vi "SPCSplitIntensityFrames.vi"(6 "New Image Size\nwhen != 0":T1={"X Size"=0, "Y Size"=0, "adc_res"=4096, "NoOfRoutingChannel"=1}, 8 "Error In":errorcluster, 9 "SPC/QC":bool=TRUE, 10 "EventData":u16[](array[numeric]) format="%04x", 11 "ROIShifts":cluster{dbl, dbl}[](array[cluster])) -> (0 "Error Out":errorcluster, 1 "IntensityFrames":cluster{u32[][]}[](array[cluster]), 2 "AbsoluteIntensity":u32[](array[numeric]), 3 "DecayMatrix":u16[][][][](array[numeric]), 4 "FrameEvents":i32[](array[numeric]), 5 "IntensityGraph":u32[][](graph), 7 "MaxIntensity":u32)   [LabVIEW 2019]
doc: "This VI goes through an EventData-Array received from 'SPC_read_fifo.vi' and interprets the events as markers or photons and populates a DecayMatrix for a single frame.\nThe 4 dimensions of DecayMatrix are the decay curves according to the microTime values of photons, in their image X- and Y-axis position and routing channel.\nNote the two possible ways of creating an IntensityGraph: With every photon event the intensity could increase per X-Y-coordinate, or the really counted photon number during a pixel event is used (usually higher).\nA functional global variable concept is used to initialize the control cluster and output arrays.\nThis VI accumulates only events for one frame.\nA similar VI used at the executable example 'ImagingEventStream-FifoImage.exe' that also collects multiple frames with improved memory management is available at B&H.\n\ninfo@becker-hickl.com"
uses:
  SPC_Controls/Fifo_CounterCluster.ctl
panel:
  out "BufferedImageSize":T1={"X Size"=0, "Y Size"=0, "adc_res"=0, "NoOfRoutingChannel"=1}
  out "CounterCluster":T2={"Pixel No"=0, "Frame No"=-1, "LastPixelTime"=0, "Line No"=-1, "StopFrame"=FALSE, "StartFrame"=FALSE, "Frame Flag"=FALSE, "Out Of Y"=FALSE, "MT-Overflow"=FALSE, "Photon Count"=0, "LineLength"=0, "FrameHeight"=0, "MT-Overflow"=0, "PixelDwellTime"=0}
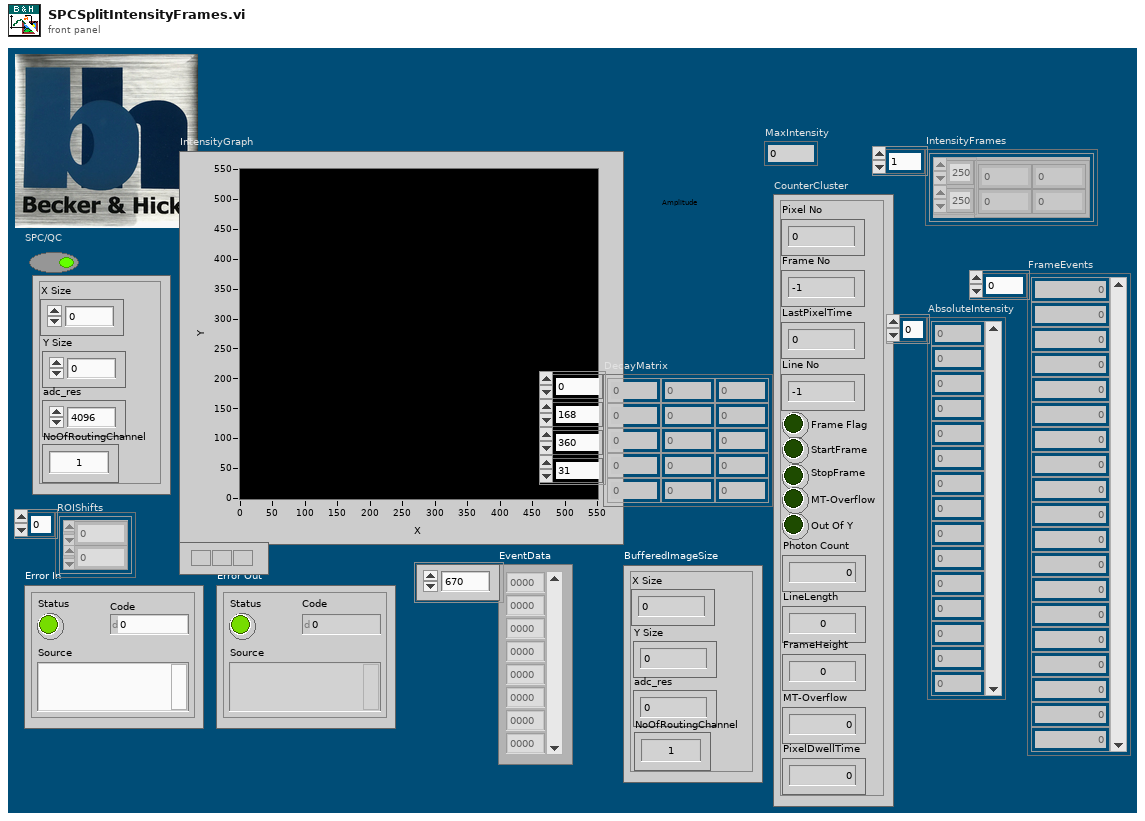
[diagram p1: front panel]
types:
  T1 = cluster{"X Size":i32, "Y Size":i32, "adc_res":i32, "NoOfRoutingChannel":i32}
  T2 = typedef "Fifo_CounterCluster.ctl" = cluster{"Pixel No":i32, "Frame No":i32, "LastPixelTime":i32, "Line No":i32, "StopFrame":bool, "StartFrame":bool, "Frame Flag":bool, "Out Of Y":bool, "MT-Overflow":bool, "Photon Count":u64, "LineLength":i32, "FrameHeight":i32, "MT-Overflow":u32, "PixelDwellTime":u32}
  T3 = cluster{"X Size":i32, "Y Size":i32, "not used":i32, "NoOfRoutingChannel":i32}
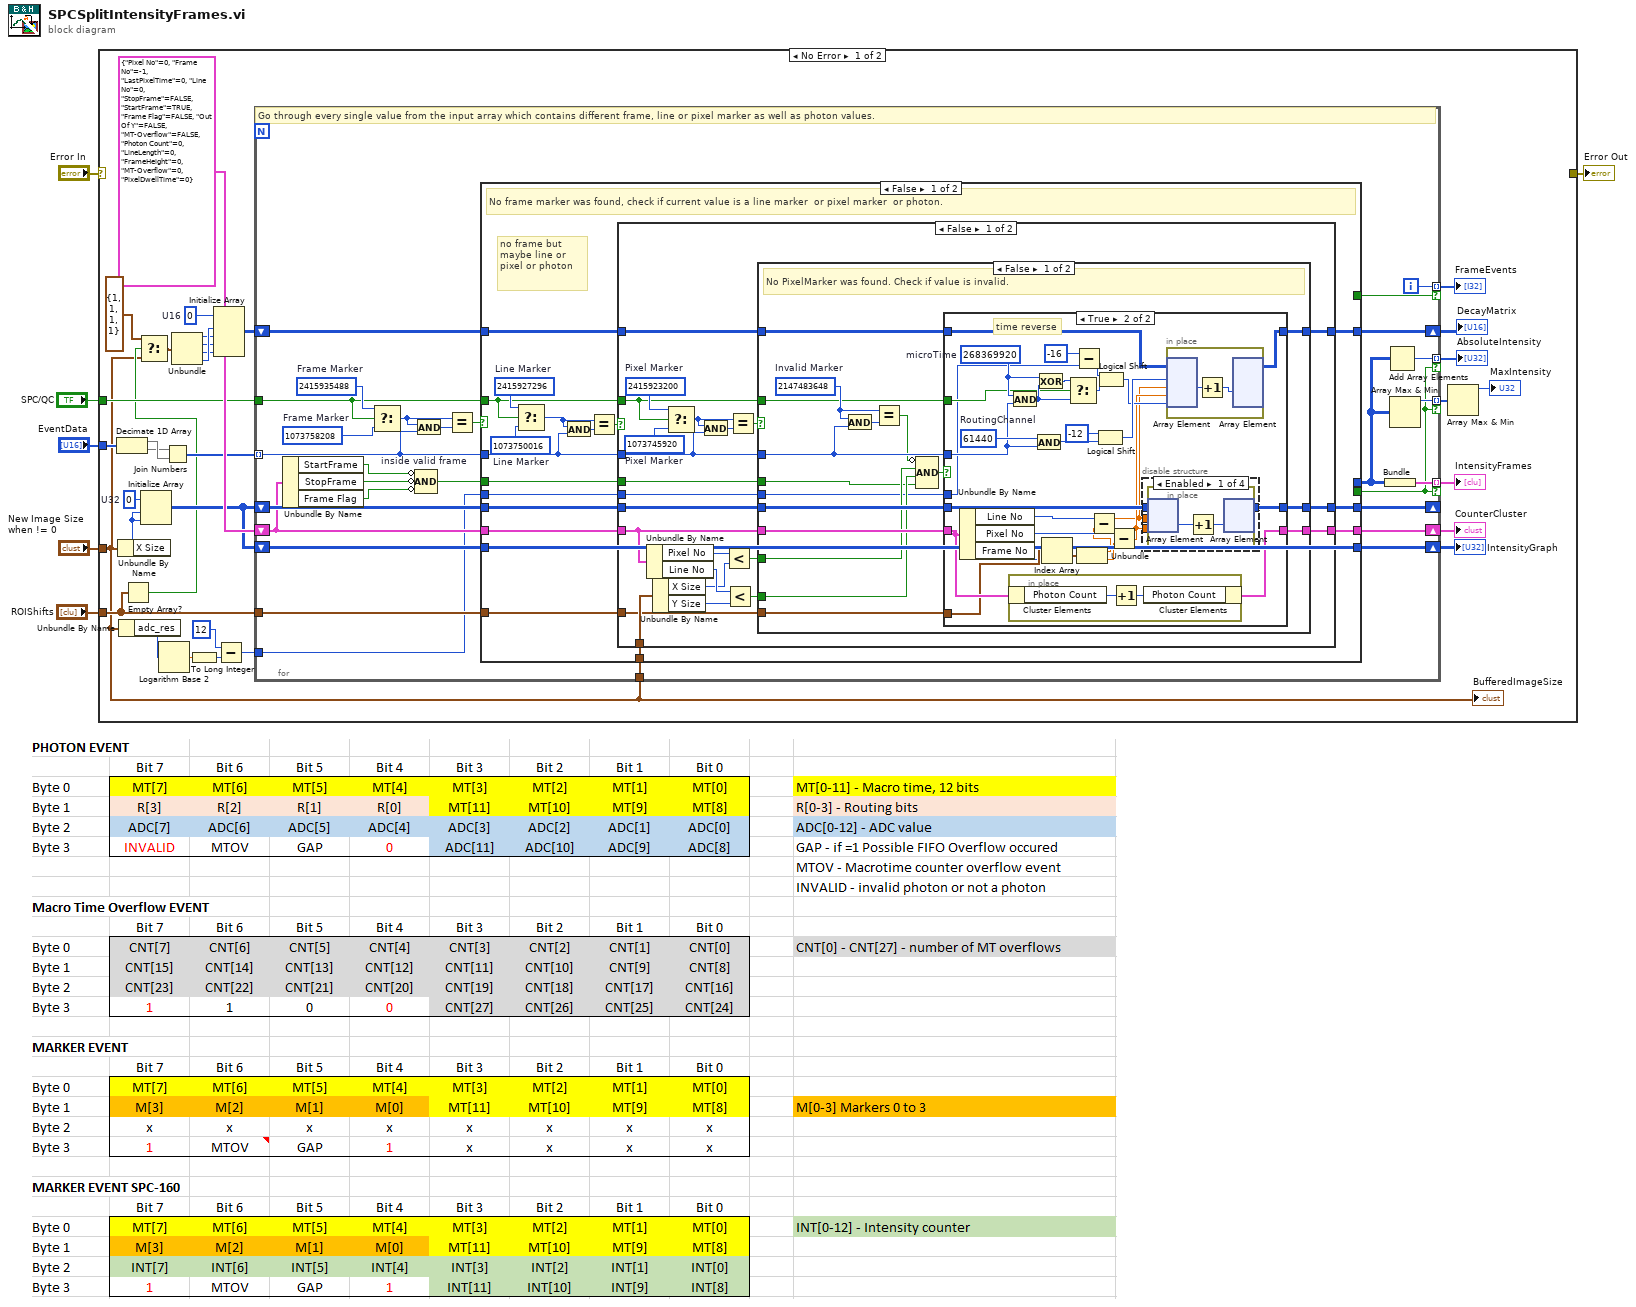
[diagram p0: block diagram]
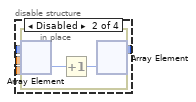
[diagram p3: hidden frame]
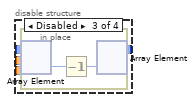
[diagram p4: hidden frame]
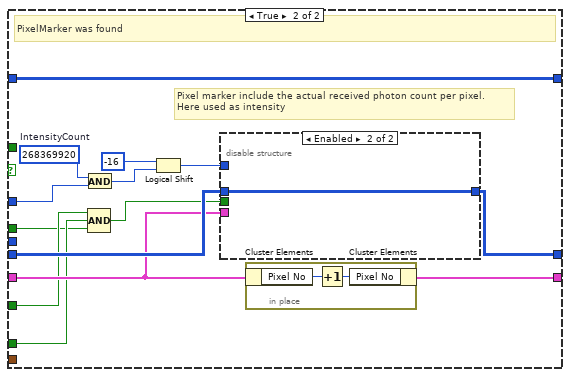
[diagram p6: hidden frame]
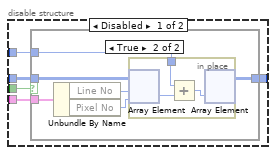
[diagram p7: hidden frame]
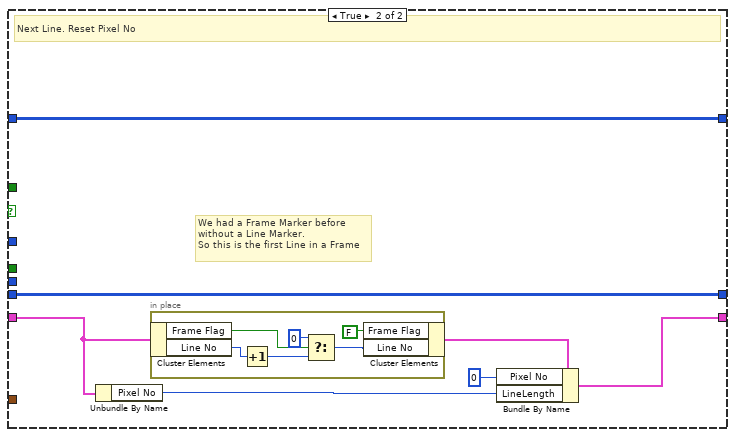
[diagram p9: hidden frame]
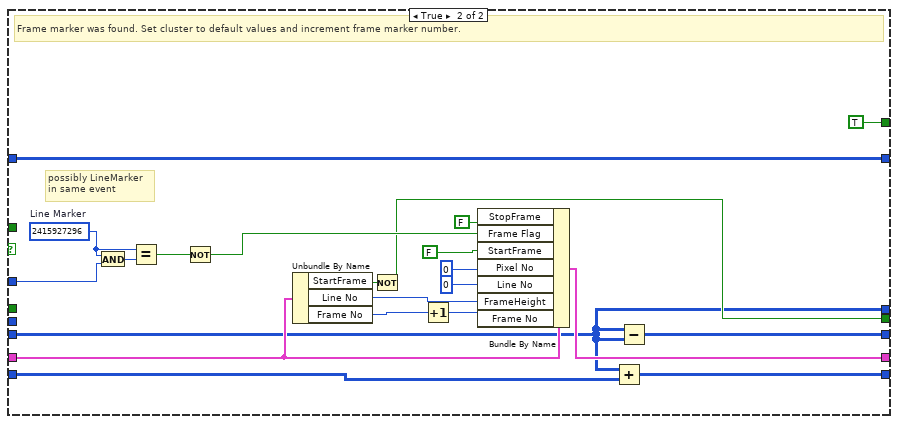
[diagram p10: hidden frame]
diagram:
  n1 = case shown="No Error" "Error In" {
    selector: "Error In" -> [_ w249]
    tunnel: [_ w249] -> w5
    tunnel: "New Image Size\nwhen != 0" -> [w9 _]
    tunnel: "EventData" -> [w39 _]
    tunnel: "SPC/QC" -> [w24 _]
    tunnel: "ROIShifts" -> [w16 _]
    frame No Error {
      w22 = u16 0  # U16
      w37 = u32 0  # U32
      n2 = Decimate 1D Array(w39) -> (w33:u16[], w32:u16[])
      n3 = Unbundle By Name(w9) -> ("X Size"=w36:i32)
      n4 = Unbundle By Name(w9) -> ("adc_res"=w8:i32)
      n5 = Empty Array?(array=w16) -> (empty?=w14:bool)
      n6 = Select(t=T3 {"X Size"=1, "Y Size"=1, "not used"=1, "NoOfRoutingChannel"=1}, s=w14, f=w9) -> (s? t:f=w15:T1)
      n7 = Initialize Array(w37, w36, w36) -> (w29:u32[][])
      n8 = Logarithm Base 2(1:w8) -> (0:w12:dbl)
      n9 = Join Numbers(hi=w32, lo=w33) -> ((hi.lo)=w34:u32[])
      n10 = Unbundle(w15) -> ("X Size"=w21:i32, "Y Size"=w20:i32, "adc_res"=w19:i32, "NoOfRoutingChannel"=w23:i32)
      n11 = To Long Integer(number=w12) -> (32bit integer=w11:i32)
      n12 = Initialize Array(w22, w23, w21, w20, w19) -> (w18:u16[][][][])
      n13 = Subtract(x=12, y=w11) -> (x-y=w7:i32)
      n14 = for {
        tunnel: w34 -> [w65] mode=indexing
        shift-right: [w68] -> w38
        shift-left: T2 {"Pixel No"=0, "Frame No"=-1, "LastPixelTime"=0, "Line No"=0, "StopFrame"=FALSE, "StartFrame"=TRUE, "Frame Flag"=FALSE, "Out Of Y"=FALSE, "MT-Overflow"=FALSE, "Photon Count"=0, "LineLength"=0, "FrameHeight"=0, "MT-Overflow"=0, "PixelDwellTime"=0} ("Counter Cluster") -> [w64]
        shift-right: [w66] -> _
        shift-left: w29 -> [w67]
        tunnel: [w57] -> w31 mode=indexing if=w49
        tunnel: w9 -> [w56]
        shift-right: [w55] -> w30
        shift-left: w29 -> [w54]
        tunnel: [w53] -> w28 mode=indexing if=w48
        tunnel: [w52] -> w27 mode=indexing if=w49
        tunnel: [w50] -> w25 mode=indexing if=w49
        tunnel: w24 -> [w44]
        shift-right: [w43] -> w17
        shift-left: w18 -> [w42]
        tunnel: w16 -> [w41]
        tunnel: w7 -> [w40]
        i -> [w53]
        w45 = u32 1073758208  # Frame Marker
        w47 = u32 2415935488  # Frame Marker
        # "Go through every single value from the input array which contains different frame, line or pixel marker as well as photon values."
        n15 = Unbundle By Name(w64) -> ("StartFrame"=w61:bool, "StopFrame"=w60:bool, "Frame Flag"=w59:bool)
        n16 = Select(t=w47, s=w44, f=w45) -> (s? t:f=w46:u32)
        n17 = And(x=w46, y=w65) -> (x .and. y?=w63:u32)
        n18 = Compound Arithmetic op=AND "inside valid frame"(invert w61, invert w60, invert w59) -> (w58:bool)
        n19 = Equal?(x=w46, y=w63) -> (x = y?=w62:bool)
        n20 = case shown="False" w62 {
          tunnel: w64 -> [w85 w245]
          tunnel: [w84 w248] -> w68
          tunnel: w65 -> [w81 w242]
          tunnel: w67 -> [w83 w231]
          tunnel: [w82 w237] -> w66
          tunnel: w58 -> [w79 _]
          tunnel: [_ w231] -> w51
          tunnel: [_ w233] -> w49
          tunnel: w56 -> [w78 _]
          tunnel: [w77 w230] -> w55
          tunnel: w54 -> [w77 w229]
          tunnel: [_ TRUE] -> w48
          tunnel: w44 -> [w73 _]
          tunnel: [w72 w227] -> w43
          tunnel: w42 -> [w71 w227]
          tunnel: w41 -> [w70 _]
          tunnel: w40 -> [w69 _]
          frame False {
            w74 = u32 1073750016  # Line Marker
            w76 = u32 2415927296  # Line Marker
            # "no frame but maybe line or pixel or photon"
            # "No frame marker was found, check if current value is a line marker  or pixel marker  or photon."
            n21 = Select(t=w76, s=w73, f=w74) -> (s? t:f=w75:u32)
            n22 = And(x=w75, y=w81) -> (x .and. y?=w86:u32)
            n23 = Equal?(x=w75, y=w86) -> (x = y?=w80:bool)
            n24 = case shown="False" w80 {
              tunnel: w85 -> [w96 w217]
              tunnel: [w108 w219] -> w84
              tunnel: w81 -> [w104 _]
              tunnel: w83 -> [w107 w218]
              tunnel: [w106 w218] -> w82
              tunnel: w78 -> [w99 _]
              tunnel: w79 -> [w95 _]
              tunnel: w73 -> [w89 _]
              tunnel: [w91 w214] -> w72
              tunnel: w71 -> [w90 w214]
              tunnel: w70 -> [w88 _]
              tunnel: w69 -> [w87 _]
              frame False {
                w92 = u32 1073745920  # Pixel Marker
                w94 = u32 2415923200  # Pixel Marker
                n25 = Unbundle By Name(w96) -> ("Pixel No"=w100:i32, "Line No"=w103:i32)
                n26 = Unbundle By Name(w99) -> ("X Size"=w101:i32, "Y Size"=w102:i32)
                n27 = Select(t=w94, s=w89, f=w92) -> (s? t:f=w93:u32)
                n28 = And(x=w93, y=w104) -> (x .and. y?=w109:u32)
                n29 = Less?(x=w100, y=w101) -> (x < y?=w97:bool)
                n30 = Less?(x=w103, y=w102) -> (x < y?=w98:bool)
                n31 = Equal?(x=w93, y=w109) -> (x = y?=w105:bool)
                n32 = case shown="False" w105 {
                  tunnel: [w124 w195] -> w108
                  tunnel: w96 -> [w123 w192]
                  tunnel: w107 -> [w126 w194]
                  tunnel: [w125 w193] -> w106
                  tunnel: w104 -> [w120 w190]
                  tunnel: w98 -> [w122 w185]
                  tunnel: w97 -> [w121 w186]
                  tunnel: w95 -> [w115 w183]
                  tunnel: [w114 w182] -> w91
                  tunnel: w90 -> [w113 w182]
                  tunnel: w89 -> [w112 _]
                  tunnel: w88 -> [w111 _]
                  tunnel: w87 -> [w110 _]
                  frame False {
                    w119 = u32 2147483648  # Invalid Marker
                    # "No PixelMarker was found. Check if value is invalid."
                    n33 = And(x=w119, y=w120) -> (x .and. y?=w118:u32)
                    n34 = Equal?(x=w119, y=w118) -> (x = y?=w117:bool)
                    n35 = Compound Arithmetic op=AND(invert w117, w121, w122, w115) -> (w116:bool)
                    n36 = case shown="True" w116 {
                      tunnel: w126 -> [w129 w158]
                      tunnel: [w129 w157] -> w125
                      tunnel: w123 -> [w128 w156]
                      tunnel: w120 -> [_ w146]
                      tunnel: [w128 w155] -> w124
                      tunnel: [w127 w148] -> w114
                      tunnel: w113 -> [w127 w147]
                      tunnel: w112 -> [_ w140]
                      tunnel: w111 -> [_ w139]
                      tunnel: w110 -> [_ w130]
                      frame False {
                      }
                      frame True {
                        w150 = u32 61440  # RoutingChannel
                        w149 = u32 268369920  # microTime
                        # "time reverse"
                        n37 = Unbundle By Name(w156) -> ("Line No"=w145:i32, "Pixel No"=w144:i32, "Frame No"=w138:i32)
                        n38 = in-place {
                          n39 = in-place-cluster #1(w156) -> ("Photon Count"=w181:u64)
                          n40 = Increment(x=w181) -> (x+1=w180:u64)
                          n41 = in-place-cluster #1("Photon Count"=w180) -> (w155:T2)
                        }
                        n42 = And(x=w149, y=w146) -> (x .and. y?=w143:u32)
                        n43 = And(x=w150, y=w146) -> (x .and. y?=w151:u32)
                        n44 = Exclusive Or(1:w143, 2:w149) -> (0:w142:u32)
                        n45 = Index Array(array=w139, index=w138) -> (element=w137:cluster{dbl, dbl})
                        n46 = Select(t=w142, s=w140, f=w143) -> (s? t:f=w141:u32)
                        n47 = Subtract(x=-16, y=w130) -> (x-y=w131:i32)
                        n48 = Unbundle(w137) -> (w133:dbl, w134:dbl)
                        n49 = Subtract(x=w145, y=w133) -> (x-y=w135:dbl)
                        n50 = Logical Shift(y=i16 -12, x=w151) -> (x << y=w154:u32)
                        n51 = Logical Shift(y=w131, x=w141) -> (x << y=w153:u32)
                        n52 = Subtract(x=w144, y=w134) -> (x-y=w136:dbl)
                        n53 = disable-structure shown="Enabled" {
                          disable-tunnel: w158 -> [w164 w170 w176 w179]
                          disable-tunnel: [w163 w169 w175 w179] -> w157
                          disable-tunnel: w135 -> [w162 w168 w174 _]
                          disable-tunnel: w136 -> [w161 w167 w173 _]
                          frame Enabled {
                            n54 = in-place {
                              n55 = in-place-array #2(w164, w162, w161) -> (w166:u32)
                              n56 = Increment(x=w166) -> (x+1=w165:u32)
                              n57 = in-place-array #2(w165) -> (w163:u32[][])  [unwired: 2 out]
                            }
                          }
                          frame Disabled {
                            n58 = in-place {
                              n59 = in-place-array #3(w170, w168, w167) -> (w172:u32)
                              n60 = Increment(x=w172) -> (x+1=w171:u32)
                              n61 = in-place-array #3(w171) -> (w169:u32[][])  [unwired: 2 out]
                            }
                          }
                          frame Disabled {
                            n62 = in-place {
                              n63 = in-place-array #4(w176, w174, w173) -> (w178:u32)
                              n64 = Decrement(x=w178) -> (x-1=w177:u32)
                              n65 = in-place-array #4(w177) -> (w175:u32[][])  [unwired: 2 out]
                            }
                          }
                          frame Disabled {
                          }
                        }
                        n66 = in-place {
                          n67 = in-place-array #5(w147, w154, w135, w136, w153) -> (w160:u16)
                          n68 = Increment(x=w160) -> (x+1=w159:u16)
                          n69 = in-place-array #5(w159) -> (w148:u16[][][][])  [unwired: 4 out]
                        }
                      }
                    }
                  }
                  frame True {
                    w191 = u32 268369920  # IntensityCount
                    # "Pixel marker include the actual received photon count per pixel.\nHere used as intensity"
                    # "PixelMarker was found"
                    n70 = And(x=w191, y=w190) -> (x .and. y?=w188:u32)
                    n71 = Compound Arithmetic op=AND(w186, w185, w183) -> (w184:bool)
                    n72 = Logical Shift(y=-16, x=w188) -> (x << y=w187:u32)
                    n73 = disable-structure shown="Enabled" {
                      disable-tunnel: w194 -> [w200 w211]
                      disable-tunnel: [w199 w211] -> w193
                      disable-tunnel: w192 -> [w198 _]
                      disable-tunnel: w187 -> [w197 _]
                      disable-tunnel: w184 -> [w196 _]
                      frame Disabled {
                        n74 = case shown="True" w196 {
                          tunnel: w200 -> [w201 w207]
                          tunnel: [w201 w206] -> w199
                          tunnel: w198 -> [_ w205]
                          tunnel: w197 -> [_ w204]
                          frame False {
                          }
                          frame True {
                            n75 = Unbundle By Name(w205) -> ("Line No"=w203:i32, "Pixel No"=w202:i32)
                            n76 = in-place {
                              in-place-border: w204 -> [w208]
                              n77 = in-place-array #6(w207, w203, w202) -> (w210:u32)
                              n78 = Add(x=w208, y=w210) -> (x+y=w209:u32)
                              n79 = in-place-array #6(w209) -> (w206:u32[][])  [unwired: 2 out]
                            }
                          }
                        }
                      }
                      frame Enabled {
                      }
                    }
                    n80 = in-place {
                      n81 = in-place-cluster #7(w192) -> ("Pixel No"=w213:i32)
                      n82 = Increment(x=w213) -> (x+1=w212:i32)
                      n83 = in-place-cluster #7("Pixel No"=w212) -> (w195:T2)
                    }
                  }
                }
              }
              frame True {
                # "We had a Frame Marker before\nwithout a Line Marker.\nSo this is the first Line in a Frame"
                # "Next Line. Reset Pixel No"
                n84 = Unbundle By Name(w217) -> ("Pixel No"=w215:i32)
                n85 = in-place {
                  n86 = in-place-cluster #8(w217) -> ("Frame Flag"=w225:bool, "Line No"=w222:i32)
                  n87 = Increment(x=w222) -> (x+1=w221:i32)
                  n88 = Select(t=0, s=w225, f=w221) -> (s? t:f=w226:i32)
                  n89 = in-place-cluster #8("Frame Flag"=FALSE, "Line No"=w226) -> (w216:T2)
                }
                n90 = Bundle By Name(cluster=w216, "Pixel No"=0, "LineLength"=w215) -> (w219:T2)
              }
            }
          }
          frame True {
            w243 = u32 2415927296  # Line Marker
            # "possibly LineMarker\nin same event"
            # "Frame marker was found. Set cluster to default values and increment frame marker number."
            n91 = And(x=w243, y=w242) -> (x .and. y?=w244:u32)
            n92 = Equal?(x=w243, y=w244) -> (x = y?=w240:bool)
            n93 = Not(x=w240) -> (.not. x?=w238:bool)
            n94 = Unbundle By Name(w245) -> ("StartFrame"=w234:bool, "Line No"=w241:i32, "Frame No"=w236:i32)
            n95 = Not(x=w234) -> (.not. x?=w233:bool)
            n96 = Increment(x=w236) -> (x+1=w232:i32)
            n97 = Bundle By Name(cluster=w245, "StopFrame"=FALSE, "Frame Flag"=w238, "StartFrame"=FALSE, "Pixel No"=0, "Line No"=0, "FrameHeight"=w241, "Frame No"=w232) -> (w248:T2)
            n98 = Add(x=w231, y=w229) -> (x+y=w230:u32[][])
            n99 = Subtract(x=w231, y=w231) -> (x-y=w237:u32[][])
          }
        }
        n100 = Bundle(w51) -> (w57:cluster{u32[][]})  [unwired: 1 in]
        n101 = Add Array Elements(numeric array=w51) -> (sum=w50:u32)
        n102 = Array Max & Min(array=w51) -> (max value=w52:u32)  [unwired: 3 out]
      }
      "CounterCluster" <- w38
      "IntensityGraph" <- w30
      "IntensityFrames" <- w31
      "FrameEvents" <- w28
      "AbsoluteIntensity" <- w25
      "DecayMatrix" <- w17
      n103 = Array Max & Min(array=w27) -> (max value=→"MaxIntensity":u32)  [unwired: 3 out]
      "BufferedImageSize" <- w9
    }
    frame Error {
    }
  }
  "Error Out" <- w5
